vi "BT_Discover.vi"() -> (3 "Active_BT_Devices":T1)   [LabVIEW 2016]
uses:
  controls/BT_Devices.ctl
panel:
  out "service list":T2(array[cluster])
  out "device list":T3(array[cluster])=[{"Address"="00:06:66:8c:9e:7d", "Device Name"="RNBT-9E7D"}, {"Address"="00:14:03:05:08:37", "Device Name"="DSD TECH HC-05"}, {"Address"="94:7b:e7:8c:64:e5", "Device Name"="Galaxy A3 (2017)"}]
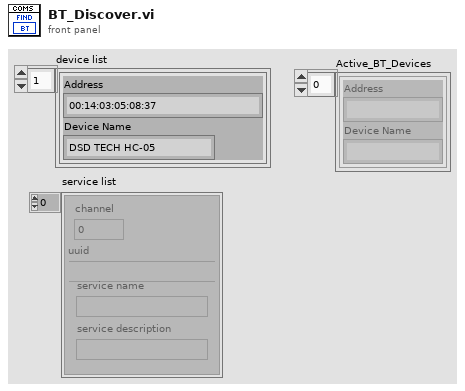
[diagram p1: front panel]
types:
  T1 = typedef "BT_Devices.ctl" = cluster{"Address":string, "Device Name":string}[]
  T2 = cluster{"channel":u16, "uuid":string, "service name":string, "service description":string}[]
  T3 = cluster{"Address":string, "Device Name":string}[]
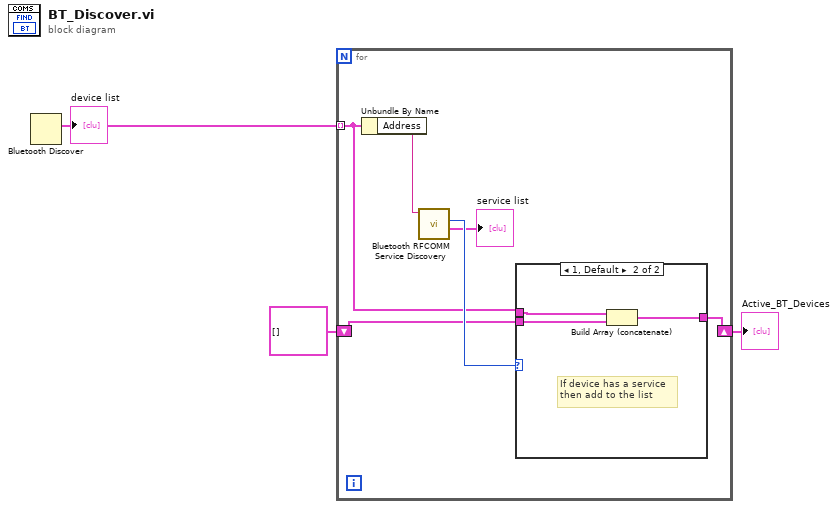
[diagram p0: block diagram]
diagram:
  n1 = Bluetooth Discover() -> (2:w3:T3)  [unwired: 2 in, 2 out]
  "device list" <- w3
  n2 = for {
    tunnel: w3 -> [w4] mode=indexing
    shift-right: [w5] -> w2
    shift-left: T3 [] -> [w6]
    n3 = Unbundle By Name(w4) -> ("Address"=w9:string)
    n4 = call <vilib>:"Bluetooth RFCOMM Service Discovery.vi"("address in"=w9) -> ("service list"=→"service list":T2, "number of services"=w8:u16)  [unwired: 3 in, 2 out]
    n5 = case shown="1, Default" w8 {
      tunnel: w4 -> [_ w13]
      tunnel: w6 -> [w10 w12]
      tunnel: [w10 w11] -> w5
      frame 0 {
      }
      frame 1, Default {
        # "If device has a service \nthen add to the list"
        n6 = Build Array (concatenate)(w13, w12) -> (w11:T3)
      }
    }
  }
  "Active_BT_Devices" <- w2
